vi "RFt Gen.vi"(9 "Seciton Num":u16, 10 "End V":dbl, 11 "Start V":dbl) -> (3 "Points":dbl[](array[numeric]))   [LabVIEW 2020, in "Actor_AFG.lvlib"]
uses:
  Actor_AFG.lvlib
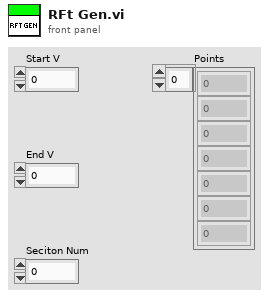
[diagram p1: front panel]
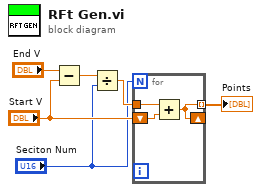
[diagram p0: block diagram]
diagram:
  n1 = Subtract(x="End V", y="Start V") -> (x-y=w2:dbl)
  n2 = Divide(x=w2, y="Seciton Num") -> (x/y=w5:dbl)
  n3 = for {
    N: "Seciton Num" -> [_]
    shift-right: [w7] -> _
    shift-left: "Start V" -> [w9]
    tunnel: w5 -> [w8]
    tunnel: [w7] -> w6 mode=indexing
    n4 = Add(x=w8, y=w9) -> (x+y=w7:dbl)
  }
  "Points" <- w6
